vi "ex_YesOrNoToBool.vi"(10 "YesOrNo String":string) -> (1 "error":bool, 2 "Yes?":bool, 3 "output string":string)   [LabVIEW 2020]
panel:
  in  "false string":string="no"
  in  "true string":string="yes"
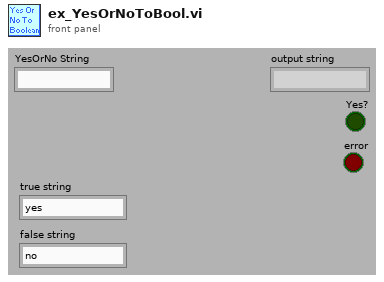
[diagram p1: front panel]
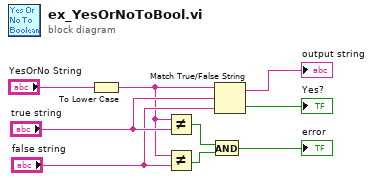
[diagram p0: block diagram]
diagram:
  n1 = To Lower Case(string="YesOrNo String") -> (all lower case string=w1:string)
  n2 = Not Equal?(x=w1, y="true string") -> (x != y?=w6:bool)
  n3 = Not Equal?(x=w1, y="false string") -> (x != y?=w5:bool)
  n4 = And(x=w6, y=w5) -> (x .and. y?=→"error":bool)
  n5 = Match True/False String(2:"false string", 3:"true string", 4:w1) -> (0:→"Yes?":bool, 1:→"output string":string)
